vi "step1 FindEdgePiece.vi"(8 "error in (no error)":errorcluster, 11 "cube in":T1) -> (0 "error out":errorcluster, 3 "cube out":T1)   [LabVIEW 2011]
doc: "Rotate cube as necessary so that the top middle piece matches the desired start colour.\n\nNo transformations are done in this VI, the operations are loaded on the the operation queue bus."
uses:
  Typedef/cube.ctl
  Typedef/face.ctl
  Typedef/operation.ctl
panel:
  out "found edge on front?":bool
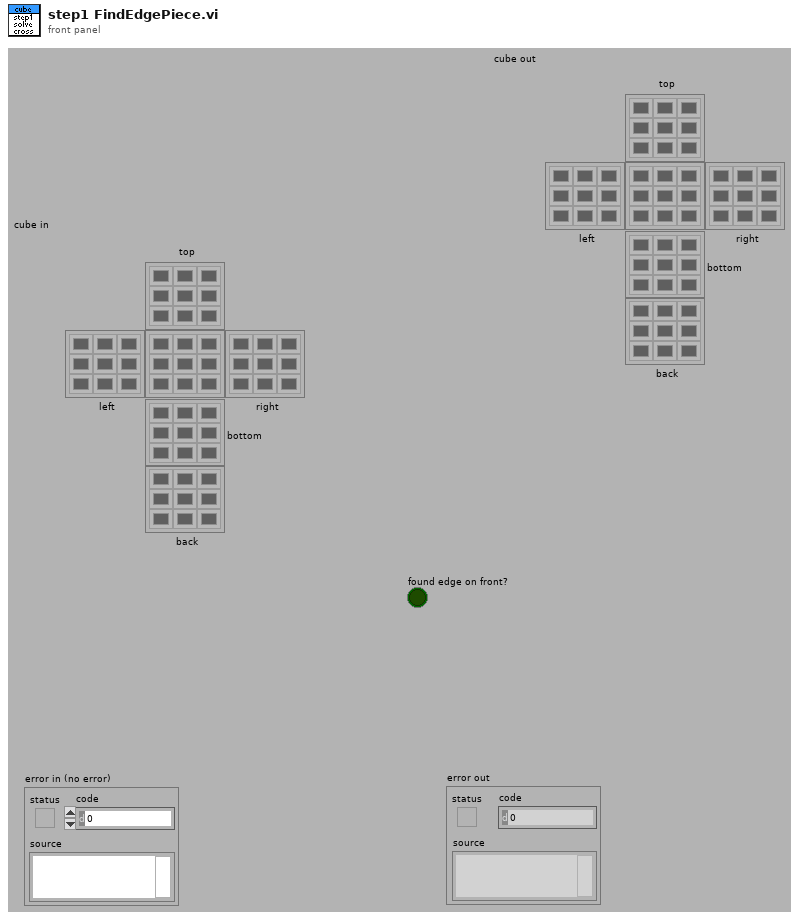
[diagram p1: front panel]
types:
  T1 = typedef "cube.ctl" = cluster{"top":T2, "left":T2, "right":T2, "bottom":T2, "back":T2, "front":T2}
  T2 = typedef "face.ctl" = u32[][]
  T3 = typedef "operation.ctl" = enum16{"nop", "T+", "T-", "F+", "F-", "L+", "L-", "R+", "R-", "B+", "B-", "<--", "-->", "^", "V"}
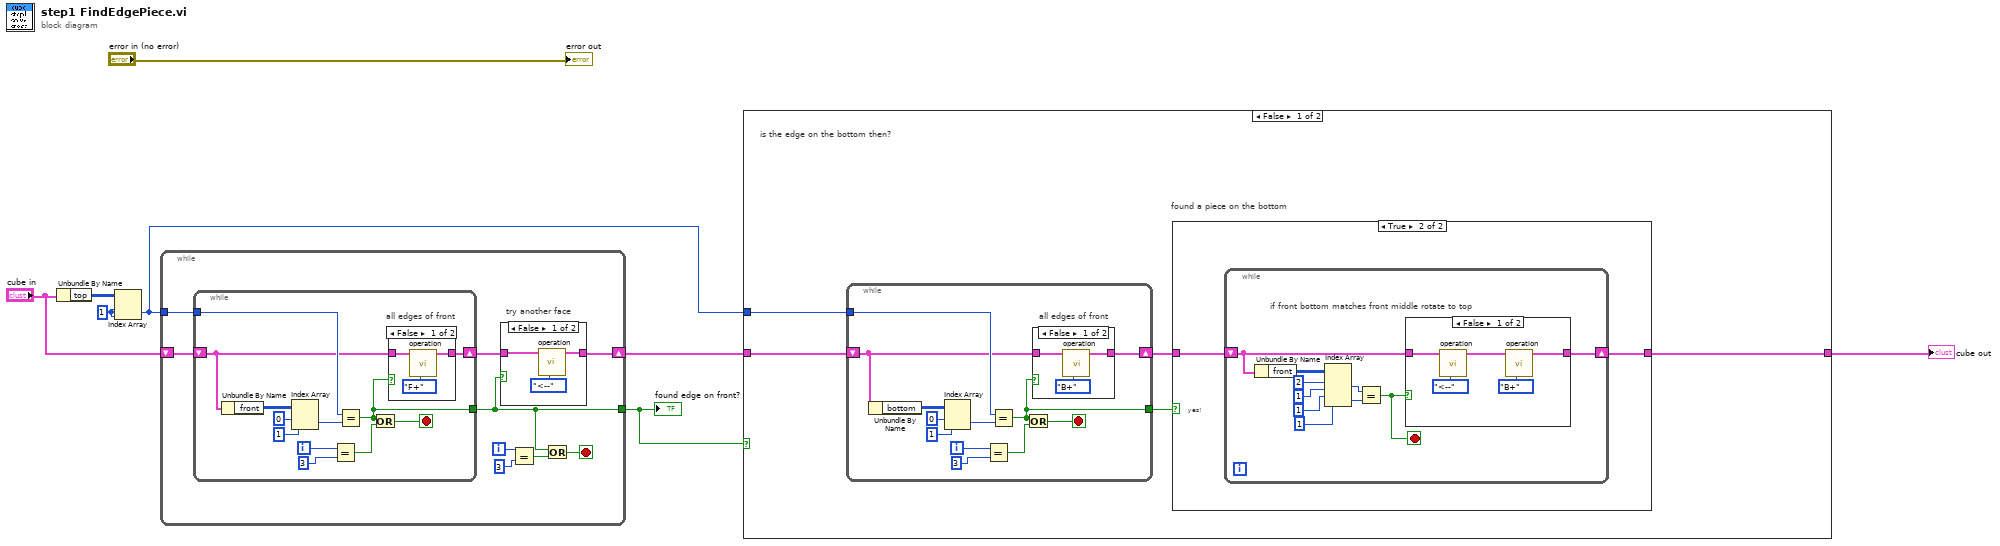
[diagram p0: block diagram]
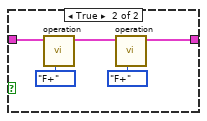
[diagram p3: hidden frame]
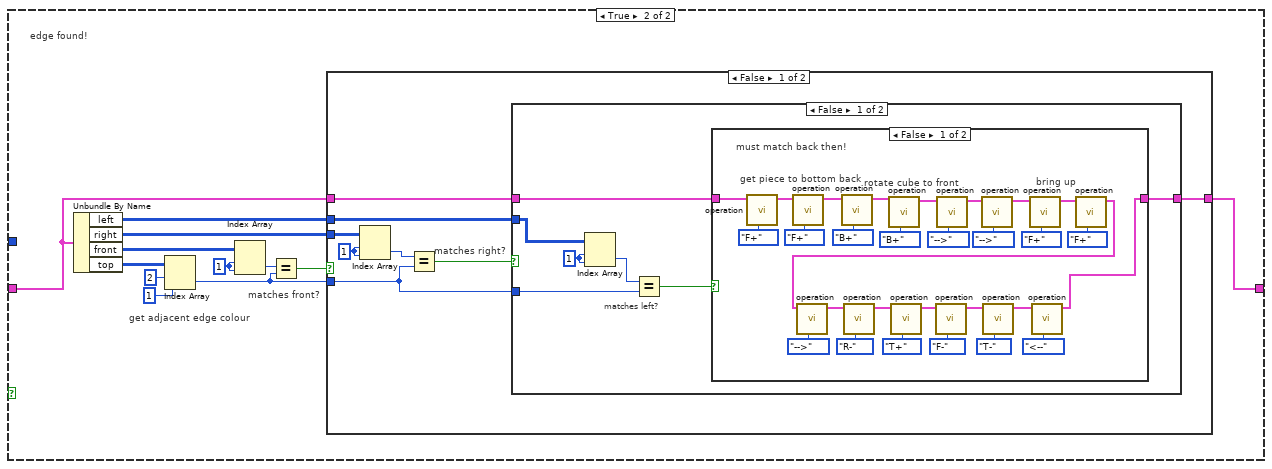
[diagram p5: hidden frame]
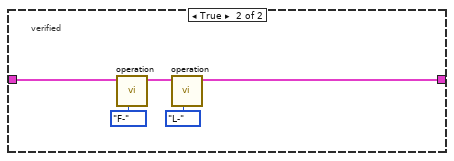
[diagram p6: hidden frame]
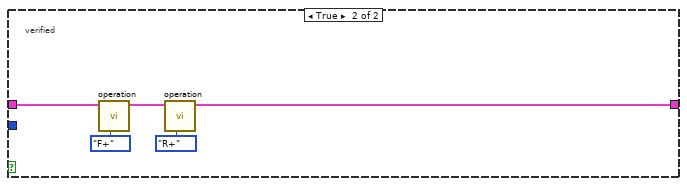
[diagram p7: hidden frame]
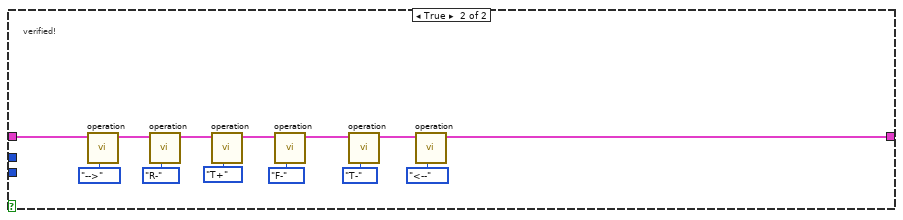
[diagram p8: hidden frame]
diagram:
  w6 = 1 ("index (row)")
  n1 = Unbundle By Name("cube in") -> ("top"=w7:T2)
  n2 = Index Array(array=w7, index (row)=w6, index (col)=w6) -> (element=w1:u32)
  n3 = while {
    tunnel: w1 -> [w17]
    tunnel: [w11] -> w3
    shift-right: [w9] -> w5
    shift-left: "cube in" -> [w15]
    i -> [w14]
    stop <- w10 stop-if-true
    # "try another face"
    n4 = while {
      tunnel: w17 -> [w31]
      shift-right: [w22] -> w16
      shift-left: w15 -> [w23]
      tunnel: [w24] -> w11
      i -> [w28]
      stop <- w25 stop-if-true
      # "all edges of front"
      n5 = Unbundle By Name(w23) -> ("front"=w29:T2)
      n6 = Index Array(array=w29, index (row)=0, index (col)=1 ("index (row)")) -> (element=w30:u32)
      n7 = Equal?(x=w28, y=3 ("index (row)")) -> (x = y?=w26:bool)
      n8 = Equal?(x=w31, y=w30) -> (x = y?=w24:bool)
      n9 = Or(x=w24, y=w26) -> (x .or. y?=w25:bool)
      n10 = case shown="False" w24 {
        tunnel: w23 -> [w35 w37]
        tunnel: [w34 w37] -> w22
        frame False {
          n11 = call "operation.vi"("operation"=operation."F+", "cube in"=w35) -> ("cube out"=w34:T1)  [unwired: 8 in, 1 out]
        }
        frame True {
        }
      }
    }
    n12 = case shown="False" w11 {
      tunnel: w16 -> [w19 w21]
      tunnel: [w18 w21] -> w9
      frame False {
        n13 = call "operation.vi"("operation"=operation."<--", "cube in"=w19) -> ("cube out"=w18:T1)  [unwired: 8 in, 1 out]
      }
      frame True {
      }
    }
    n14 = Equal?(x=w14, y=3 ("index (row)")) -> (x = y?=w12:bool)
    n15 = Or(x=w11, y=w12) -> (x .or. y?=w10:bool)
  }
  "found edge on front?" <- w3
  n16 = case shown="False" w3 {
    tunnel: w5 -> [w42 w84]
    tunnel: [w38 w82] -> w2
    tunnel: w1 -> [w41 _]
    frame False {
      # "found a piece on the bottom"
      # "is the edge on the bottom then?"
      n17 = while {
        tunnel: w41 -> [w75]
        shift-right: [w66] -> w39
        shift-left: w42 -> [w67]
        tunnel: [w68] -> w40
        i -> [w72]
        stop <- w69 stop-if-true
        # "all edges of front"
        n18 = Unbundle By Name(w67) -> ("bottom"=w73:T2)
        n19 = Index Array(array=w73, index (row)=0, index (col)=1 ("index (row)")) -> (element=w74:u32)
        n20 = Equal?(x=w72, y=3 ("index (row)")) -> (x = y?=w70:bool)
        n21 = Equal?(x=w75, y=w74) -> (x = y?=w68:bool)
        n22 = Or(x=w68, y=w70) -> (x .or. y?=w69:bool)
        n23 = case shown="False" w68 {
          tunnel: w67 -> [w78 w81]
          tunnel: [w79 w81] -> w66
          frame False {
            n24 = call "operation.vi"("operation"=operation."B+", "cube in"=w78) -> ("cube out"=w79:T1)  [unwired: 8 in, 1 out]
          }
          frame True {
          }
        }
      }
      n25 = case shown="True" w40 {
        tunnel: w39 -> [w43 w44]
        tunnel: [w43 w45] -> w38
        frame False {
        }
        frame True {
          # "yes!"
          n26 = while {
            shift-right: [w47] -> w45
            shift-left: w44 -> [w46]
            stop <- w48 stop-if-true
            # "if front bottom matches front middle rotate to top"
            n27 = Unbundle By Name(w46) -> ("front"=w55:T2)
            n28 = Index Array(array=w55, index (row) #1=2 ("index (row)"), index (col) #1=1 ("index (row)"), index (row) #2=1 ("index (row)"), index (col) #2=1 ("index (row)")) -> (element #1=w50:u32, element #2=w49:u32)
            n29 = Equal?(x=w50, y=w49) -> (x = y?=w48:bool)
            n30 = case shown="False" w48 {
              tunnel: [w56 w61] -> w47
              tunnel: w46 -> [w59 w64]
              frame False {
                n31 = call "operation.vi"("operation"=operation."<--", "cube in"=w59) -> ("cube out"=w57:T1)  [unwired: 8 in, 1 out]
                n32 = call "operation.vi"("operation"=operation."B+", "cube in"=w57) -> ("cube out"=w56:T1)  [unwired: 8 in, 1 out]
              }
              frame True {
                n33 = call "operation.vi"("operation"=operation."F+", "cube in"=w64) -> ("cube out"=w62:T1)  [unwired: 8 in, 1 out]
                n34 = call "operation.vi"("operation"=operation."F+", "cube in"=w62) -> ("cube out"=w61:T1)  [unwired: 8 in, 1 out]
              }
            }
          }
        }
      }
    }
    frame True {
      w88 = 1 ("index (row)")
      # "edge found!"
      # "matches front?"
      # "get adjacent edge colour"
      n35 = Unbundle By Name(w84) -> ("left"=w89:T2, "right"=w90:T2, "front"=w87:T2, "top"=w92:T2)
      n36 = Index Array(array=w92, index (row)=2, index (col)=1 ("disabled index (col)")) -> (element=w85:u32)
      n37 = Index Array(array=w87, index (row)=w88, index (col)=w88) -> (element=w86:u32)
      n38 = Equal?(x=w86, y=w85) -> (x = y?=w83:bool)
      n39 = case shown="False" w83 {
        tunnel: w90 -> [w101 _]
        tunnel: w89 -> [w97 _]
        tunnel: w85 -> [w96 _]
        tunnel: w84 -> [w95 w154]
        tunnel: [w94 w148] -> w82
        frame False {
          w100 = 1 ("index (row)")
          # "matches right?"
          n40 = Index Array(array=w101, index (row)=w100, index (col)=w100) -> (element=w99:u32)
          n41 = Equal?(x=w99, y=w96) -> (x = y?=w98:bool)
          n42 = case shown="False" w98 {
            tunnel: w97 -> [w106 _]
            tunnel: w96 -> [w105 _]
            tunnel: w95 -> [w103 w145]
            tunnel: [w102 w143] -> w94
            frame False {
              w107 = 1 ("index (row)")
              # "matches left?"
              n43 = Index Array(array=w106, index (row)=w107, index (col)=w107) -> (element=w108:u32)
              n44 = Equal?(x=w108, y=w105) -> (x = y?=w104:bool)
              n45 = case shown="False" w104 {
                tunnel: w103 -> [w110 w140]
                tunnel: [w126 w138] -> w102
                frame False {
                  # "bring up"
                  # "rotate cube to front"
                  # "get piece to bottom back"
                  # "must match back then!"
                  n46 = call "operation.vi"("operation"=operation."F+", "cube in"=w110) -> ("cube out"=w113:T1)  [unwired: 8 in, 1 out]
                  n47 = call "operation.vi"("operation"=operation."F+", "cube in"=w113) -> ("cube out"=w123:T1)  [unwired: 8 in, 1 out]
                  n48 = call "operation.vi"("operation"=operation."B+", "cube in"=w123) -> ("cube out"=w124:T1)  [unwired: 8 in, 1 out]
                  n49 = call "operation.vi"("operation"=operation."B+", "cube in"=w124) -> ("cube out"=w125:T1)  [unwired: 8 in, 1 out]
                  n50 = call "operation.vi"("operation"=operation."-->", "cube in"=w125) -> ("cube out"=w118:T1)  [unwired: 8 in, 1 out]
                  n51 = call "operation.vi"("operation"=operation."-->", "cube in"=w118) -> ("cube out"=w122:T1)  [unwired: 8 in, 1 out]
                  n52 = call "operation.vi"("operation"=operation."F+", "cube in"=w122) -> ("cube out"=w119:T1)  [unwired: 8 in, 1 out]
                  n53 = call "operation.vi"("operation"=operation."F+", "cube in"=w119) -> ("cube out"=w109:T1)  [unwired: 8 in, 1 out]
                  n54 = call "operation.vi"("operation"=operation."-->", "cube in"=w109) -> ("cube out"=w129:T1)  [unwired: 8 in, 1 out]
                  n55 = call "operation.vi"("operation"=operation."R-", "cube in"=w129) -> ("cube out"=w131:T1)  [unwired: 8 in, 1 out]
                  n56 = call "operation.vi"("operation"=operation."T+", "cube in"=w131) -> ("cube out"=w133:T1)  [unwired: 8 in, 1 out]
                  n57 = call "operation.vi"("operation"=operation."F-", "cube in"=w133) -> ("cube out"=w135:T1)  [unwired: 8 in, 1 out]
                  n58 = call "operation.vi"("operation"=operation."T-", "cube in"=w135) -> ("cube out"=w137:T1)  [unwired: 8 in, 1 out]
                  n59 = call "operation.vi"("operation"=operation."<--", "cube in"=w137) -> ("cube out"=w126:T1)  [unwired: 8 in, 1 out]
                }
                frame True {
                  # "verified"
                  n60 = call "operation.vi"("operation"=operation."F-", "cube in"=w140) -> ("cube out"=w139:T1)  [unwired: 8 in, 1 out]
                  n61 = call "operation.vi"("operation"=operation."L-", "cube in"=w139) -> ("cube out"=w138:T1)  [unwired: 8 in, 1 out]
                }
              }
            }
            frame True {
              # "verified"
              n62 = call "operation.vi"("operation"=operation."F+", "cube in"=w145) -> ("cube out"=w144:T1)  [unwired: 8 in, 1 out]
              n63 = call "operation.vi"("operation"=operation."R+", "cube in"=w144) -> ("cube out"=w143:T1)  [unwired: 8 in, 1 out]
            }
          }
        }
        frame True {
          # "verified!"
          n64 = call "operation.vi"("operation"=operation."-->", "cube in"=w154) -> ("cube out"=w153:T1)  [unwired: 8 in, 1 out]
          n65 = call "operation.vi"("operation"=operation."R-", "cube in"=w153) -> ("cube out"=w152:T1)  [unwired: 8 in, 1 out]
          n66 = call "operation.vi"("operation"=operation."T+", "cube in"=w152) -> ("cube out"=w151:T1)  [unwired: 8 in, 1 out]
          n67 = call "operation.vi"("operation"=operation."F-", "cube in"=w151) -> ("cube out"=w150:T1)  [unwired: 8 in, 1 out]
          n68 = call "operation.vi"("operation"=operation."T-", "cube in"=w150) -> ("cube out"=w149:T1)  [unwired: 8 in, 1 out]
          n69 = call "operation.vi"("operation"=operation."<--", "cube in"=w149) -> ("cube out"=w148:T1)  [unwired: 8 in, 1 out]
        }
      }
    }
  }
  "cube out" <- w2
  "error out" <- "error in (no error)"
